vi "Wait On Timer Example.vi"() -> ()   [LabVIEW 2011]
panel:
  out "Running":bool
  in  "Time":dbl=10.0 format="%.3f"
  out "Timer Value":dbl format="%.3f"
  # "This VI will run for the amount of time specified in\nby Time."
  # "Timer Value shows a running\ndisplay of the timers value"
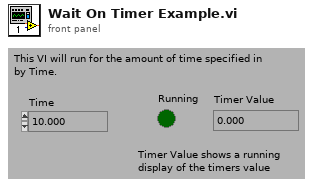
[diagram p1: front panel]
types:
  T1 = typedef "Timer Refnum.ctl" = refnum<k1>
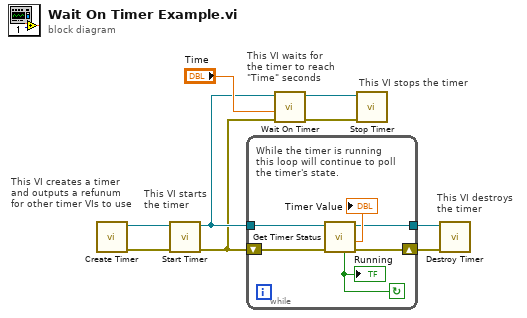
[diagram p0: block diagram]
diagram:
  # "This VI destroys\nthe timer"
  # "This VI starts\nthe timer"
  # "This VI creates a timer\nand outputs a refunum\nfor other timer VIs to use"
  # "This VI waits for\nthe timer to reach\n\"Time\" seconds"
  # "This VI stops the timer"
  n1 = call "Create Timer.vi"() -> ("error out"=w6:errorcluster, "timer"=w7:T1)  [unwired: 5 in, 1 out]
  n2 = call "Start Timer.vi"("error in (no error)"=w6, "timer"=w7) -> ("error out"=w3:errorcluster, "timer out"=w4:T1)  [unwired: 8 in]
  n3 = while {
    tunnel: [w10] -> w8
    shift-left: w3 -> [w14]
    shift-right: [w11] -> w9
    tunnel: w4 -> [w15]
    stop <- w13 continue-if-true
    # "While the timer is running\nthis loop will continue to poll\nthe timer's state."
    n4 = call "Get Timer Status.vi"("error in (no error)"=w14, "timer"=w15) -> ("error out"=w11:errorcluster, "Total time (s)"=→"Timer Value":dbl, "timer out"=w10:T1, "Running"=w13:bool)  [unwired: 4 in, 2 out]
    "Running" <- w13
  }
  n5 = call "Wait On Timer.vi"("error in (no error)"=w3, "timer value to wait for in seconds"="Time", "timer"=w4) -> ("error out"=w1:errorcluster, "timer out"=w2:T1)  [unwired: 2 in, 1 out]
  n6 = call "Stop Timer.vi"("error in (no error)"=w1, "timer"=w2) -> ()  [unwired: 8 in, 2 out]
  n7 = call "Destroy Timer.vi"("error in (no error)"=w9, "timer"=w8) -> ()  [unwired: 4 in, 2 out]
